vi "ICM Trim Whitespace.vi"(0 "string":string, 1 "location (both)":T1 items=["both", "start of string", "end of string"]) -> (2 "trimmed string":string)   [LabVIEW 2024]
doc: "Removes all white space (spaces, tabs, carriage returns, and linefeeds) from the beginning, end, or both ends of <B>string</B>."
uses:
  ICM whitespace.ctl
panel:
  # "This is a copy of an NI sub-vi. It is necessary to include it in\nthe OSDS directories so that it can be found by dynamically-called\nparsers."
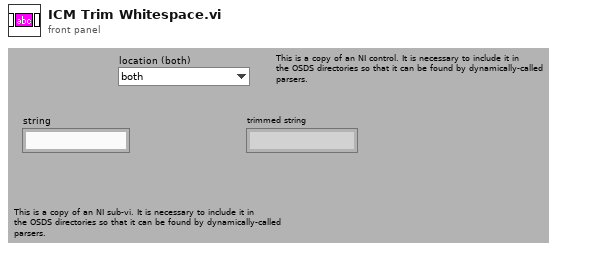
[diagram p1: front panel]
types:
  T1 = typedef "ICM whitespace.ctl" = u16
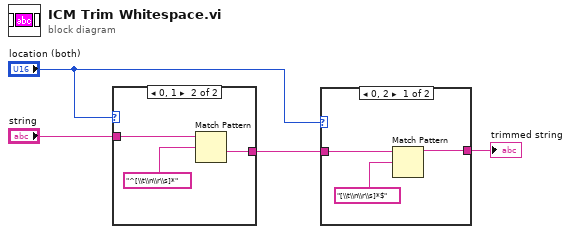
[diagram p0: block diagram]
diagram:
  n1 = case shown="0, 1" "location (both)" {
    tunnel: [w5 w8] -> w3
    tunnel: "string" -> [w5 w6]
    frame Default {
    }
    frame 0, 1 {
      n2 = Match Pattern(string=w6, regular expression="^[\\t\\n\\r\\s]*") -> (after substring=w8:string)  [unwired: 4 out]
    }
  }
  n3 = case shown="0, 2" "location (both)" {
    tunnel: [w11 w12] -> w4
    tunnel: w3 -> [w10 w12]
    frame 0, 2 {
      n4 = Match Pattern(string=w10, regular expression="[\\t\\n\\r\\s]*$") -> (before substring=w11:string)  [unwired: 4 out]
    }
    frame Default {
    }
  }
  "trimmed string" <- w4
